vi "Handle Commands.vi"(10 "FormulaG API in":refnum<class "FormulaG API.lvclass">, 11 "Cmd Q":refnum<queue>) -> (2 "FormulaG API":refnum<class "FormulaG API.lvclass">, 5 "Reset":bool)   [LabVIEW 2024, in "FormulaG.lvlib" / "FormulaG App.lvclass"]
uses:
  FormulaG App.lvclass
  Command/Command.lvclass
  FormulaG API/FormulaG API.lvclass
  Reset Cmd/Reset Cmd.lvclass
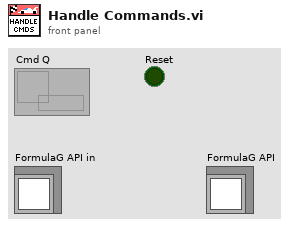
[diagram p1: front panel]
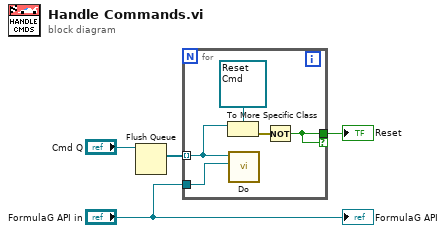
[diagram p0: block diagram]
diagram:
  n1 = Flush Queue(queue="Cmd Q") -> (remaining elements=w3:refnum<class "Command.lvclass">[])  [unwired: 1 in, 2 out]
  n2 = for {
    tunnel: w3 -> [w8] mode=indexing
    tunnel: "FormulaG API in" -> [w9]
    tunnel: [w5] -> w1 if=w5
    n3 = To More Specific Class(target class=refnum<class "Reset Cmd.lvclass"> refnum ("FormulaG.lvlib:Reset Cmd.lvclass"), reference=w8) -> (error out=w6:errorcluster)  [unwired: 1 in, 1 out]
    n4 = call-dynamic "Do.vi"("FormulaG API"=w9, "Command in"=w8) -> ()  [unwired: 8 in, 2 out]
    n5 = Not(x=w6) -> (.not. x?=w5:bool)
  }
  "Reset" <- w1
  "FormulaG API" <- "FormulaG API in"
